vi "intensity_calibration.vi"(4 "Horizontal Pixel Size 2":dbl, 5 "Control Camera Properties":T1={"Packet Size"=1500, "Pixel Format"=17825797, "Gain in dB"=1.0, "Exposure Time in µs"=1500, "Stream Bytes per Second"=50000000} {"Stream Bytes per Second" min=1000000 max=124000000 step=100000 format="%.1p"; "Exposure Time in µs" min=21 max=153391689 format="%#.0f"; "Gain in dB" min=0.0 max=26.0 format="%#_2g"; "Pixel Format" items=["Mono 12 Packed"=17563654, "Mono 12"=17825797]}, 6 "Vertical Pixel Size 2":dbl, 7 "array in":u16[][](array[numeric]), 9 "reference":refnum<vi>, 10 "appended path":path=path "C:/Users/loa/Documents/imaging-spectrometer/imaging-spectrometer/data_intensity_calibration/IC.txt", 11 "Boolean":bool) -> (2 "array out":u16[][](array[numeric]))   [LabVIEW 2014]
uses:
  type definitions/control camera properties.ctl
  <vilib>/Utility/file.llb/Read From Spreadsheet File (DBL).vi
panel:
  out "Array":dbl[][](array[numeric]) format="%#_6p"
  # "Bytes"
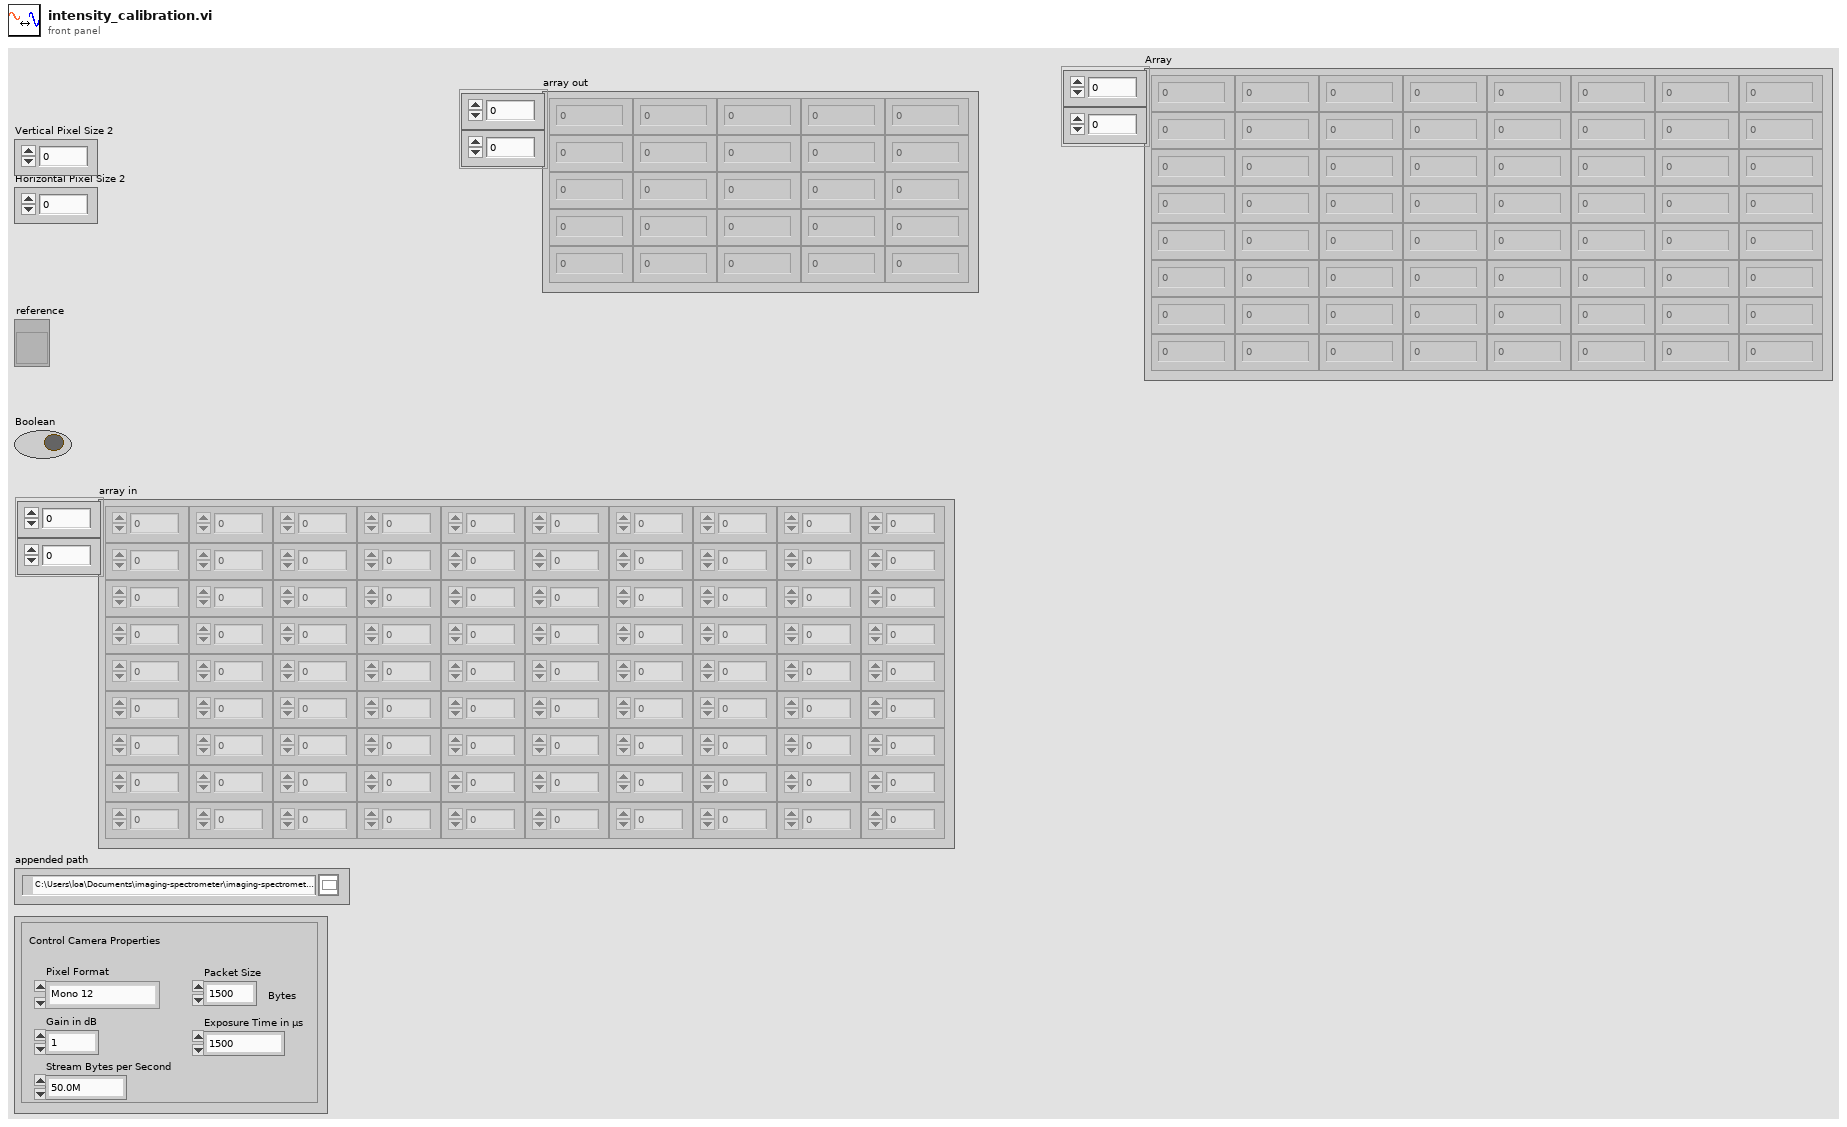
[diagram p1: front panel]
types:
  T1 = typedef "control camera properties.ctl" = cluster{"Packet Size":u32, "Pixel Format":u32, "Gain in dB":dbl, "Exposure Time in µs":u32, "Stream Bytes per Second":u32}
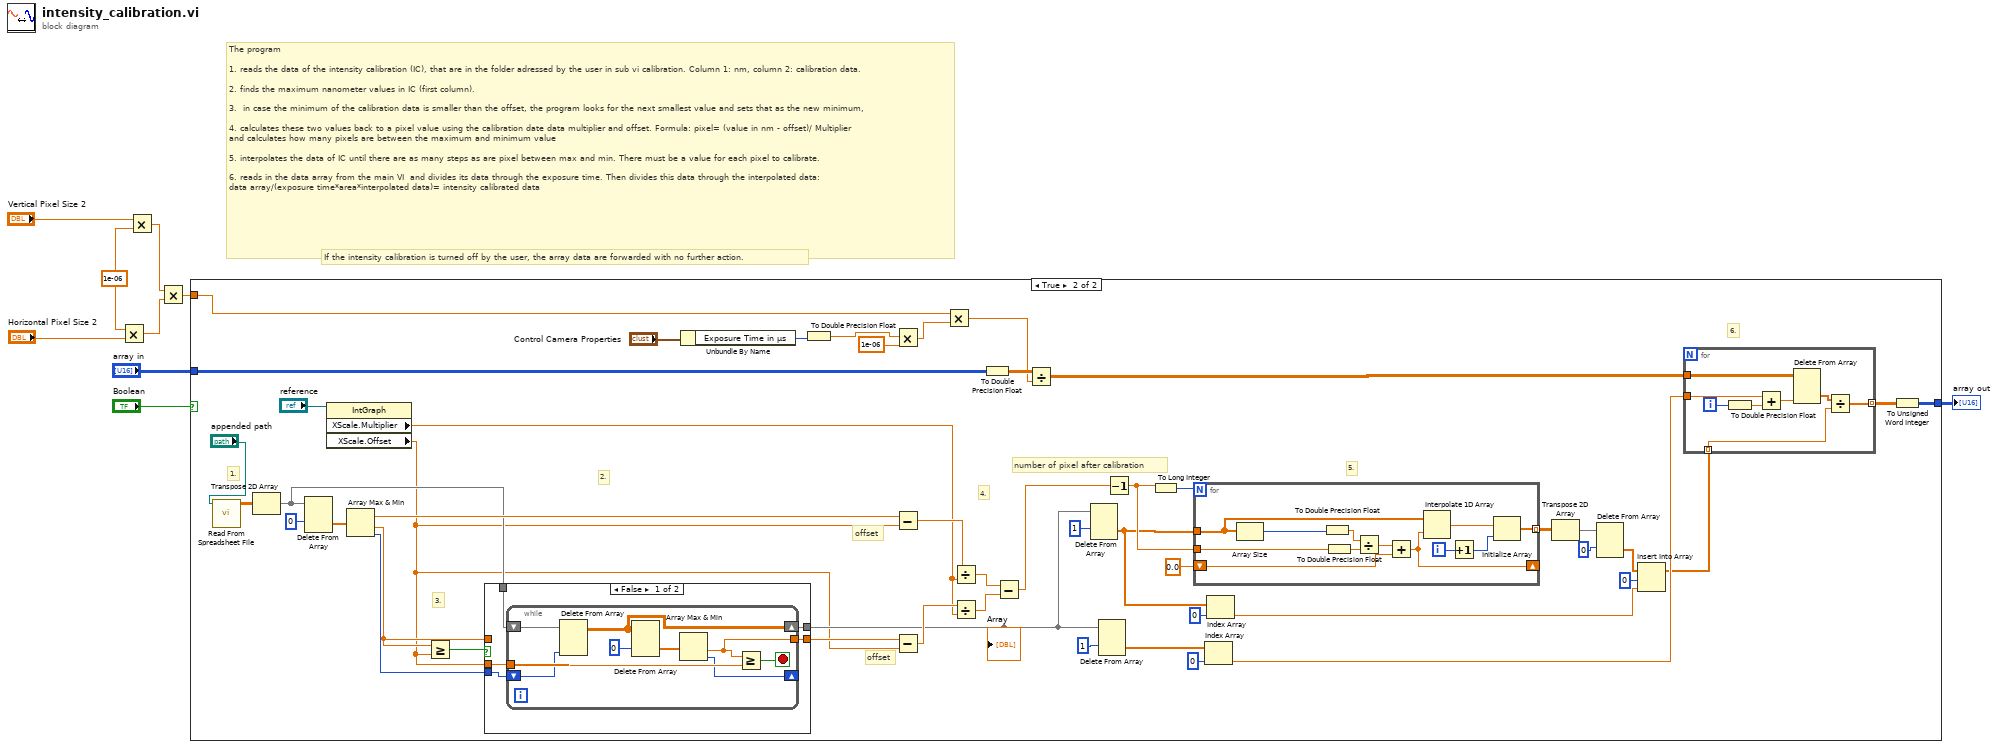
[diagram p0: block diagram]
diagram:
  w1 = 1e-06 ("y")
  # "If the intensity calibration is turned off by the user, the array data are forwarded with no further action."
  # "The program\n\n1. reads the data of the intensity calibration (IC), that are in the folder adressed by the user in sub vi calibration. Column 1: nm, column 2: calibration data.\n\n2. finds the maximum nanometer values in IC (first column). \n\n3.  in case the minimum of the calibration data is smaller than the offset, the program looks for the next smallest value and sets that as the new minimum,\n\n4. calculates these two values back to a pixel value using the calibration date data multiplier and offset. Formula: pixel= (value in nm - offset)/ Multiplier\nand calculates how many pixels are between the maximum and minimum value\n\n5. interpolates the data of IC until there are as many steps as are pixel between max and min. There must be a value for each pixel to calibrate.\n\n6. reads in the data array from the main VI  and divides its data through the exposure time. Then divides this data through the interpolated data:\ndata array/(exposure time*area*interpolated data)= intensity calibrated data"
  n1 = Multiply(x=w1, y="Horizontal Pixel Size 2") -> (x*y=w3:dbl)
  n2 = Multiply(x="Vertical Pixel Size 2", y=w1) -> (x*y=w4:dbl)
  n3 = Multiply(x=w4, y=w3) -> (x*y=w6:dbl)
  n4 = case shown="True" "Boolean" {
    tunnel: "array in" -> [w10 w22]
    tunnel: [w10 w24] -> w7
    tunnel: w6 -> [_ w16]
    frame False {
    }
    frame True {
      # "offset"
      # "offset"
      # "6."
      # "number of pixel after calibration"
      # "4."
      # "5."
      # "1."
      # "3."
      # "2."
      n5 = call-poly <vilib>:"Read From Spreadsheet File.vi"("file path (dialog if empty)"="appended path") -> ("all rows"=w57:dbl[][])  [unwired: 6 in, 4 out]
      n6 = Transpose 2D Array(2D array=w57) -> (transposed array=w46:dbl[][])
      n7 = Delete From Array(array=w46, index (row)=0) -> (deleted portion=w50:dbl[])  [unwired: 2 in, 1 out]
      n8 = property on="Property Node" class="IntGraph"(reference="reference") -> ("XScale.Multiplier"=w19:dbl, "XScale.Offset"=w18:dbl)  [unwired: 1 in, 2 out]
      n9 = Array Max & Min(array=w50) -> (max value=w56:dbl, min value=w51:dbl, min index (indices)=w49:i32)  [unwired: 1 out]
      n10 = Greater Or Equal?(x=w51, y=w18) -> (x >= y?=w52:bool)
      n11 = case shown="False" w52 {
        tunnel: w51 -> [_ w94]
        tunnel: w46 -> [w83 w93]
        tunnel: w49 -> [w82 _]
        tunnel: w18 -> [w81 _]
        tunnel: [w79 w94] -> w47
        tunnel: [w80 w93] -> w30
        frame False {
          n12 = while {
            tunnel: w81 -> [w91]
            shift-right: [w86] -> _
            shift-left: w82 -> [w90]
            shift-right: [w85] -> w80
            shift-left: w83 -> [w89]
            tunnel: [w84] -> w79
            stop <- w92 stop-if-true
            n13 = Delete From Array(array=w89, index (col)=w90) -> (array with subset deleted=w85:dbl[][])  [unwired: 2 in, 1 out]
            n14 = Delete From Array(array=w85, index (row)=0) -> (deleted portion=w87:dbl[])  [unwired: 2 in, 1 out]
            n15 = Array Max & Min(array=w87) -> (min value=w84:dbl, min index (indices)=w86:i32)  [unwired: 2 out]
            n16 = Greater Or Equal?(x=w84, y=w91) -> (x >= y?=w92:bool)
          }
        }
        frame True {
        }
      }
      "Array" <- w30
      n17 = Unbundle By Name("Control Camera Properties") -> ("Exposure Time in µs"=w21:u32)
      n18 = To Double Precision Float(number=w21) -> (double precision float=w12:dbl)
      n19 = Multiply(x=w12, y=1e-06) -> (x*y=w11:dbl)
      n20 = Subtract(x=w56, y=w18) -> (x-y=w55:dbl)
      n21 = Subtract(x=w47, y=w18) -> (x-y=w48:dbl)
      n22 = Multiply(x=w16, y=w11) -> (x*y=w15:dbl)
      n23 = Divide(x=w55, y=w19) -> (x/y=w53:dbl)
      n24 = Divide(x=w48, y=w19) -> (x/y=w54:dbl)
      n25 = To Double Precision Float(number=w22) -> (double precision float=w23:dbl[][])
      n26 = Subtract(x=w53, y=w54) -> (x-y=w42:dbl)
      n27 = Divide(x=w23, y=w15) -> (x/y=w26:dbl[][])
      n28 = Delete From Array(array=w30, index (row)=1) -> (deleted portion=w35:dbl[])  [unwired: 2 in, 1 out]
      n29 = Delete From Array(array=w30, index (row)=1) -> (deleted portion=w29:dbl[])  [unwired: 2 in, 1 out]
      n30 = Decrement(x=w42) -> (x-1=w40:dbl)
      n31 = To Long Integer(number=w40) -> (32bit integer=w41:i32)
      n32 = for {
        N: w41 -> [_]
        tunnel: w35 -> [w69]
        tunnel: [w76] -> w43 mode=indexing
        shift-right: [w68] -> _
        shift-left: 0.0 -> [w74]
        tunnel: w40 -> [w67]
        i -> [w77]
        n33 = Array Size(array=w69) -> (size(s)=w72:i32)
        n34 = To Double Precision Float(number=w72) -> (double precision float=w73:dbl)
        n35 = To Double Precision Float(number=w67) -> (double precision float=w71:dbl)
        n36 = Divide(x=w73, y=w71) -> (x/y=w75:dbl)
        n37 = Add(x=w75, y=w74) -> (x+y=w68:dbl)
        n38 = Interpolate 1D Array(1:w68, 2:w69) -> (0:w78:dbl)
        n39 = Increment(x=w77) -> (x+1=w70:i32)
        n40 = Initialize Array(w78, w70) -> (w76:dbl[])
      }
      n41 = Index Array(array=w29, index=0) -> (element=w28:dbl)
      n42 = Index Array(array=w35, index=0) -> (element=w33:dbl)
      n43 = Transpose 2D Array(2D array=w43) -> (transposed array=w36:dbl[][])
      n44 = Delete From Array(array=w36, index (row)=0) -> (deleted portion=w37:dbl[])  [unwired: 2 in, 1 out]
      n45 = Insert Into Array(array=w37, index=0, new element=w33) -> (w27:dbl[])
      n46 = for {
        tunnel: w26 -> [w66]
        tunnel: w27 -> [w63] mode=indexing
        tunnel: [w64] -> w25 mode=indexing
        tunnel: w28 -> [w62]
        i -> [w60]
        n47 = To Double Precision Float(number=w60) -> (double precision float=w59:dbl)
        n48 = Add(x=w62, y=w59) -> (x+y=w61:dbl)
        n49 = Delete From Array(array=w66, index (col)=w61) -> (deleted portion=w65:dbl[])  [unwired: 2 in, 1 out]
        n50 = Divide(x=w65, y=w63) -> (x/y=w64:dbl[])
      }
      n51 = To Unsigned Word Integer(number=w25) -> (unsigned 16bit integer=w24:u16[][])
    }
  }
  "array out" <- w7
